vi "InsertSession.vi"(5 "connection reference":T1, 6 "session_start_time":timestamp, 7 "session_path":path, 8 "error in (no error)":errorcluster, 9 "experimenter":string, 10 "subject":string, 11 "setup":u8) -> (0 "error out":errorcluster, 3 "SessionPK":T2)   [LabVIEW 2014]
uses:
  <vilib>/addons/database/NI_Database_API.lvlib
  SessionPrimary.ctl
  <vilib>/addons/database/Connection.llb/Conn ObjectReference.ctl
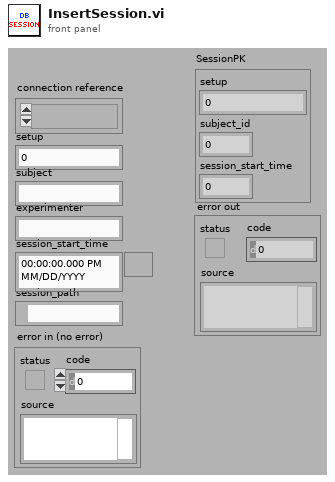
[diagram p1: front panel]
types:
  T1 = typedef "NI_Database_API.lvlib/Conn ObjectReference.ctl" = refnum<k1>
  T2 = typedef "SessionPrimary.ctl" = cluster{"setup":u8, "subject_id":i32, "session_start_time":dbl}
  T3 = cluster{"setup":u8, "subject":string, "experimenter":string, "session_start_time":timestamp, "session_path":path}
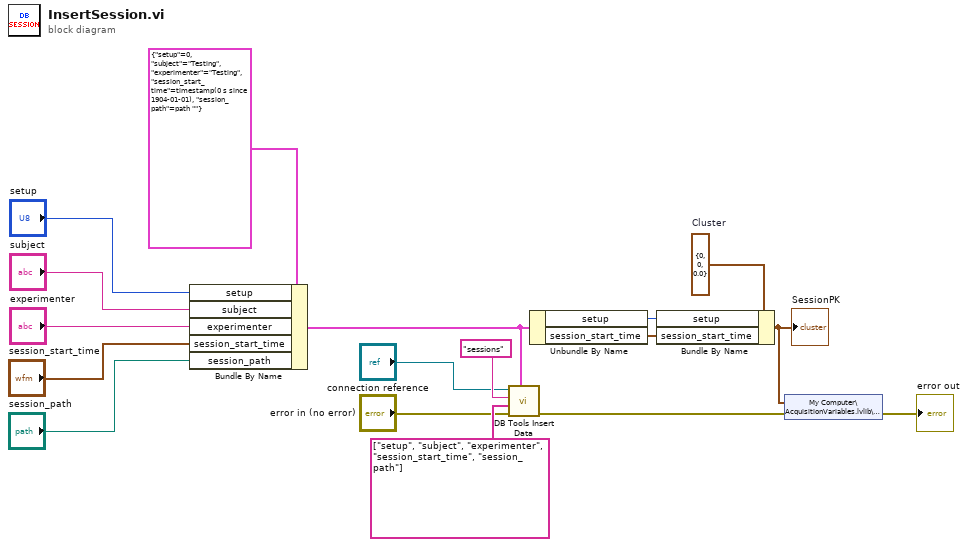
[diagram p0: block diagram]
diagram:
  w9 = T2 {"setup"=0, "subject_id"=0, "session_start_time"=0.0}  # Cluster
  n1 = Bundle By Name(cluster=T3 {"setup"=0, "subject"="Testing", "experimenter"="Testing", "session_start_time"=timestamp(0 s since 1904-01-01), "session_path"=path ""} ("Cluster"), "setup"="setup", "subject"="subject", "experimenter"="experimenter", "session_start_time"="session_start_time", "session_path"="session_path") -> (w8:T3)
  n2 = call <vilib>:"DB Tools Insert Data.vi"("data"=w8, "error in (no error)"="error in (no error)", "columns"=string[] ["setup", "subject", "experimenter", "session_start_time", "session_path"], "table"="sessions", "connection reference"="connection reference") -> ("error out"=w2:errorcluster)  [unwired: 5 in, 1 out]
  n3 = Unbundle By Name(w8) -> ("setup"=w7:u8, "session_start_time"=w6:timestamp)
  n4 = Bundle By Name(cluster=w9, "setup"=w7, "session_start_time"=w6) -> (w3:T2)
  "SessionPK" <- w3
  n5 = shared-variable "My Computer\\AcquisitionVariables.lvlib\\SessionPK"(w3, error in=w2) -> (error out=→"error out":errorcluster)
